vi "zadanie2_kol.vi"() -> ()   [LabVIEW 2012]
panel:
  in  "stop":bool
  out "XY Graph":cluster{"Y":dbl[], "Y":dbl[]}[](graph)
  in  "faza sygnału generator 2":dbl(knob) scale=0.0..360.0
  in  "faza sygnału generator 1":dbl(knob) scale=0.0..360.0
  in  "Częstotliwość generator 2":dbl
  in  "Amplituda generator 2":dbl
  in  "Częstotliwość generator 1":dbl
  in  "Amplituda generator 1":dbl
  # "Program dokonuje pomiaru różnicy fazy dwóch generatorów i przedstawia na wykresie\nna podstawie usawionej przez użytkownika amplitudy, częstotliwości i fazy sygnału"
  # "generator 1"
  # "generator 2"
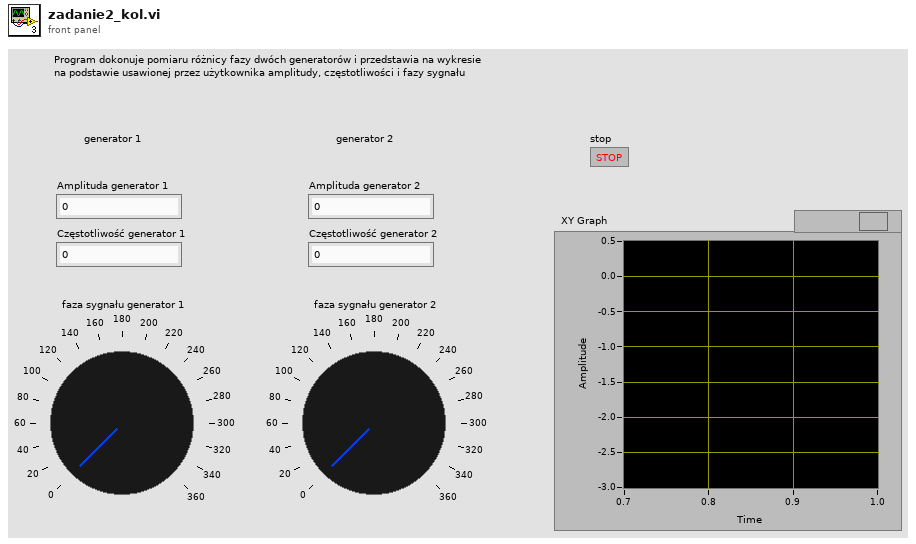
[diagram p1: front panel]
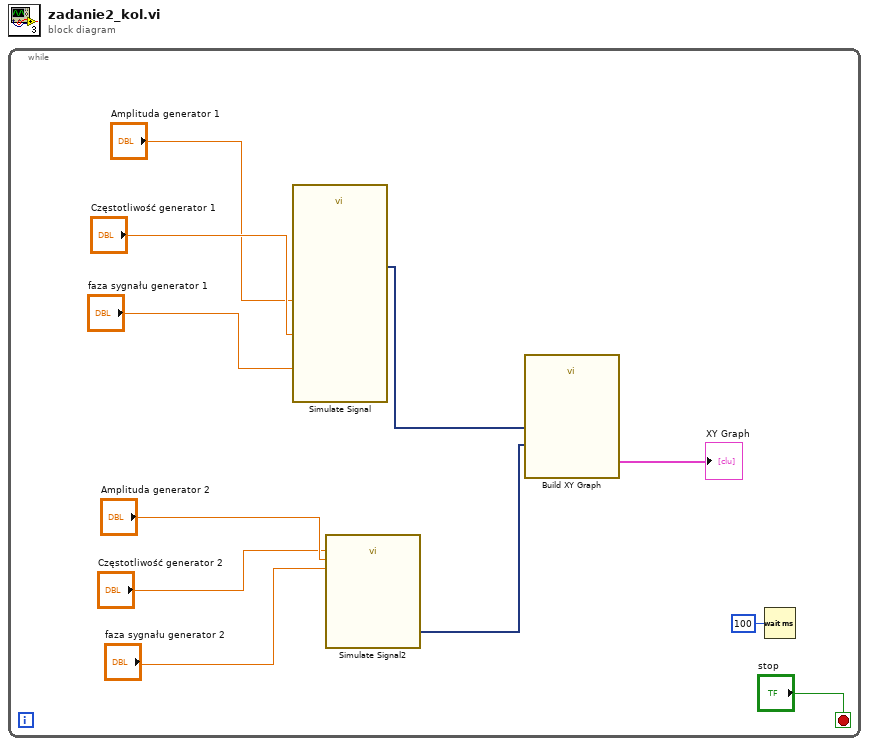
[diagram p0: block diagram]
diagram:
  n1 = while {
    stop <- "stop" stop-if-true
    n2 = call "Simulate Signal"("Frequency"="Częstotliwość generator 1", "Amplitude"="Amplituda generator 1", "Phase"="faza sygnału generator 1") -> ("Sine one"=w1:dynamicdata)  [unwired: 11 in, 1 out]
    n3 = call "Simulate Signal2"("Frequency"="Częstotliwość generator 2", "Amplitude"="Amplituda generator 2", "Phase"="faza sygnału generator 2") -> ("Sine one"=w2:dynamicdata)  [unwired: 11 in, 1 out]
    n4 = call "Build XY Graph"("Y Input"=w2, "X Input"=w1) -> ("XY Graph"=→"XY Graph":cluster{"Y":dbl[], "Y":dbl[]}[])  [unwired: 3 in, 6 out]
    n5 = Wait (ms)(milliseconds to wait=u32 100) -> ()  [unwired: 1 out]
  }
